vi "Put Raw Wrapper.vi"(8 "error in (no error)":errorcluster, 9 "Raw Data":u8[](array[numeric]) format="%.0x", 10 "key":string="myhome/kitchen/temp", 11 "Session in":u64) -> (0 "error out":errorcluster)   [LabVIEW 2021, in "Zenoh.lvclass"]
uses:
  Zenoh.lvclass
  Zenoh.lvclass/Zenoh.ctl
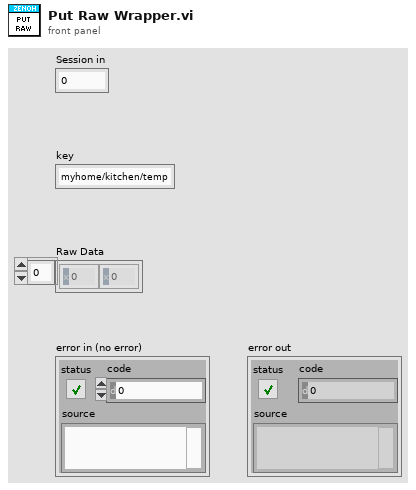
[diagram p1: front panel]
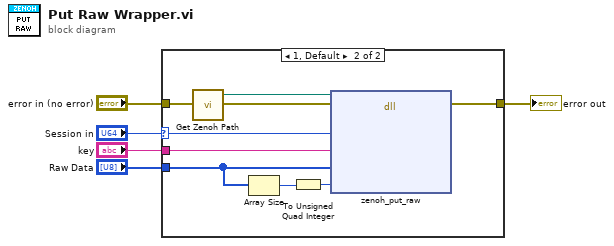
[diagram p0: block diagram]
diagram:
  n1 = case shown="1, Default" "Session in" {
    selector: "Session in" -> [_ w12]
    tunnel: [w6 w7] -> w5
    tunnel: "error in (no error)" -> [w6 w13]
    tunnel: "key" -> [_ w11]
    tunnel: "Raw Data" -> [_ w10]
    frame 0 {
    }
    frame 1, Default {
      n2 = call "Get Zenoh Path.vi"() -> ("Library Path"=w14:path)  [unwired: 4 in]
      n3 = Array Size(array=w10) -> (size(s)=w9:i32)
      n4 = To Unsigned Quad Integer(1:w9) -> (0:w8:u64)
      n5 = dll-call lib="C:/Program Files/CIF_Foundation/Libraries/zenoh_lv_wrapper.dll" fn="zenoh_put_raw" label="ZenohPut Raw"(path in=w14, error in=w13, "session_ptr"=w12, "key"=w11, "data"=w10, "data_len"=w8) -> (error out=w7:errorcluster)  [unwired: 6 in, 1 out]
    }
  }
  "error out" <- w5
